vi "Begin.vi"() -> (0 "error out":errorcluster)   [LabVIEW 2013]
doc: "Called before other user functions, this VI is expected to open initial I/O refnums, load in file data, and do all program initialization. Notice that the <B>error out</B> terminal is simply used for data flow. Wiring it to other structures or subVIs ensures that this VI runs first."
uses:
  <vilib>/Rock Robotics/WPI/DriverStation/WPI_DriverStationRobotMode2.ctl
  <vilib>/Rock Robotics/WPI/Joystick/WPI_JoystickDeviceEnum.ctl
  <vilib>/Rock Robotics/SystemInterfaces/DIO/FPGA_DIOPWMChannel.ctl
  <vilib>/Rock Robotics/SystemInterfaces/DIO/FPGA_DIOChannel.ctl
  <vilib>/Rock Robotics/SystemInterfaces/Typedef/FPGA_TypedefDigitalModule.ctl
  Robot Global Data.vi
  <vilib>/Rock Robotics/WPI/RobotDrive/WPI_RobotDriveOpen4MotorWithVictor.vi
  <vilib>/Rock Robotics/WPI/Counter/WPI_CounterDigitalInputToDigitalSource.vi
  <vilib>/Rock Robotics/WPI/Counter/WPI_CounterOpen UpDown Mode.vi
  <vilib>/Rock Robotics/WPI/MotorControl/WPI_MotorControlOpen Victor.vi
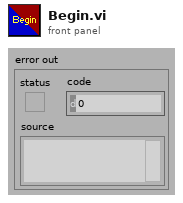
[diagram p1: front panel]
types:
  T1 = typedef "FPGA_DIOPWMChannel.ctl" = enum8{"PWM 1", "PWM 2", "PWM 3", "PWM 4", "PWM 5", "PWM 6", "PWM 7", "PWM 8", "PWM 9", "PWM 10", "Invalid"}
  T2 = typedef "FPGA_TypedefDigitalModule.ctl" = enum16{"Digital Module 1", "Digital Module 2"}
  T3 = typedef "FPGA_DIOChannel.ctl" = enum8{"DIO 1", "DIO 2", "DIO 3", "DIO 4", "DIO 5", "DIO 6", "DIO 7", "DIO 8", "DIO 9", "DIO 10", "DIO 11", "DIO 12", "DIO 13", "DIO 14", "Invalid"}
  T4 = typedef "WPI_JoystickDeviceEnum.ctl" = enum16{"USB 1", "USB 2", "USB 3", "USB 4", "Kinect 1", "Kinect 2"}
  T5 = typedef "WPI_DriverStationRobotMode2.ctl" = enum16{"Autonomous Disabled", "Autonomous Enabled", "Teleop Disabled", "Teleop Enabled", "Timeout", "Finish", "Test Disabled", "Test Enabled"}
  T6 = typedef "WPI_JoystickDevRef.ctl" = cluster{"Device":T4}
  T7 = typedef "WPI_DigitalInputDevRef.ctl" = cluster{"DevStatus":errorcluster, "DIO Channel":T3, "Digital Module":T2}
  T8 = typedef "WPI_MotorControlDeviceRef.ctl" = cluster{"DeviceStatus":errorcluster, "Type":enum16{"PWM", "CAN"}, "PWM":cluster{"Digital Module":T2, "PWM Channel":T1, "DeadBand":T9}, "CAN":cluster{"Device Number":u8, "Control Mode":T10, "Semaphore":T11, "Max Vout":dbl}, "Invert":bool, "TransformRef":T12, "InvTransformRef":T12}
  T9 = typedef "WPI_PWMDeadband.ctl" = cluster{"Name":string, "maxPositivePwm":i32, "minPositivePwm":i32, "centerPwm":i32, "maxNegativePwm":i32, "minNegativePwm":i32, "angularRange":u16}
  T10 = typedef "WPI_CANJaguar_ControlMode.ctl" = enum8{"Percent VBus", "Current", "Speed", "Position", "Voltage"}
  T11 = typedef "Semaphore RefNum" = refnum<k1>
  T12 = typedef "WPI_PWMTransform_ConPane.ctl" = refnum<vi>
  T13 = typedef "WPI_RobotDriveDevRef.ctl" = cluster{"DevStatus":errorcluster, "Motors[]":T8[], "Square Inputs":bool, "Max Output":dbl, "Isochronous":bool}
  T14 = typedef "FPGA_CounterEncoderSourceConvertionLVSourceType.ctl" = cluster{"DevStatus":errorcluster, "AnalogTriggerMode?":bool, "DigitalMode":cluster{"Digital Module":T2, "DIO Channel":T15}, "AnalogTriggerMode":cluster{"AnalogTriggerIndex":T16, "OutputType":T17}}
  T15 = typedef "FPGA_DIODigitalSourceChannel.ctl" = enum8{"DIO 1", "DIO 2", "DIO 3", "DIO 4", "DIO 5", "DIO 6", "DIO 7", "DIO 8", "DIO 9", "DIO 10", "DIO 11", "DIO 12", "DIO 13", "DIO 14", "Disabled"}
  T16 = typedef "FPGA_AnalogTriggerIndex.ctl" = enum8{"Trig 0", "Trig 1", "Trig 2", "Trig 3", "Trig 4", "Trig 5", "Trig 6", "Trig 7", "Invalid"}
  T17 = typedef "FPGA_AnalogTriggerOutType.ctl" = enum16{"InWindow", "TriggerState", "Rising", "Falling"}
  T18 = typedef "WPI_CounterDevRef.ctl" = cluster{"DevStatus":errorcluster, "CntIndex":T19}
  T19 = typedef "FPGA_CounterCtrSystemIndex.ctl" = enum8{"Ctr 0", "Ctr 1", "Ctr 2", "Ctr 3", "Ctr 4", "Ctr 5", "Ctr 6", "Ctr 7", "Invalid"}
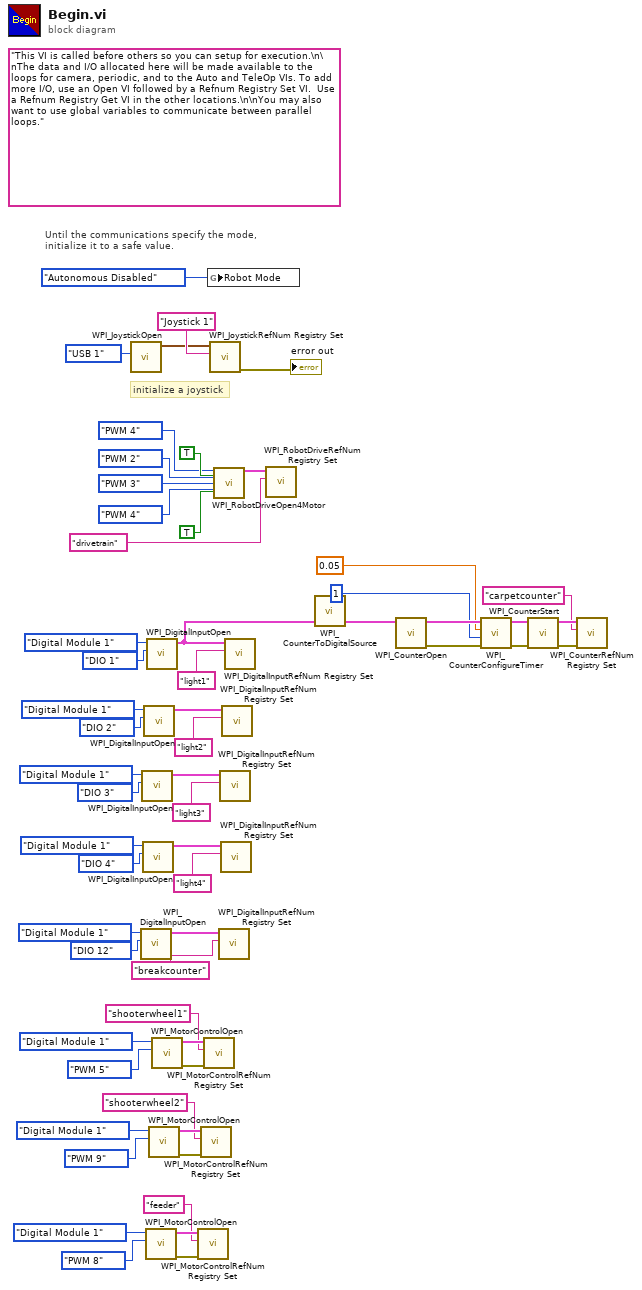
[diagram p0: block diagram]
diagram:
  (unwired) "This VI is called before others so you can setup for execution.\n\nThe data and I/O allocated here will be made available to the loops for camera, periodic, and to the Auto and TeleOp VIs. To add more I/O, use an Open VI followed by a Refnum Registry Set VI.  Use a Refnum Registry Get VI in the other locations.\n\nYou may also want to use global variables to communicate between parallel loops."
  # "initialize a joystick"
  # "Until the communications specify the mode,\ninitialize it to a safe value."
  n1 = call <vilib>:"WPI_JoystickOpen.vi"("JoystickDevice"=WPI_JoystickDeviceEnum."USB 1") -> ("JoystickDevRef"=w56:T6)  [unwired: 10 in]
  n2 = call <vilib>:"WPI_DigitalInputOpen.vi"("DIO Channel"=FPGA_DIOChannel."DIO 12", "Digital Module (Module 1)"=FPGA_TypedefDigitalModule."Digital Module 1") -> ("DigitalInputDevRef"=w30:T7)  [unwired: 8 in, 1 out]
  n3 = call <vilib>:"WPI_DigitalInputOpen.vi"("DIO Channel"=FPGA_DIOChannel."DIO 3", "Digital Module (Module 1)"=FPGA_TypedefDigitalModule."Digital Module 1") -> ("DigitalInputDevRef"=w38:T7)  [unwired: 8 in, 1 out]
  n4 = call <vilib>:"WPI_DigitalInputOpen.vi"("DIO Channel"=FPGA_DIOChannel."DIO 4", "Digital Module (Module 1)"=FPGA_TypedefDigitalModule."Digital Module 1") -> ("DigitalInputDevRef"=w34:T7)  [unwired: 8 in, 1 out]
  n5 = call <vilib>:"WPI_DigitalInputOpen.vi"("DIO Channel"=FPGA_DIOChannel."DIO 2", "Digital Module (Module 1)"=FPGA_TypedefDigitalModule."Digital Module 1") -> ("DigitalInputDevRef"=w42:T7)  [unwired: 8 in, 1 out]
  n6 = call-poly <vilib>:"WPI_MotorControlOpen.vi"("PWM Channel"=FPGA_DIOPWMChannel."PWM 8", "Digital Module (Module 1)"=FPGA_TypedefDigitalModule."Digital Module 1") -> ("error out"=w4:errorcluster, "MotorControlDeviceRef"=w5:T8)  [unwired: 8 in]
  n7 = call <vilib>:"WPI_DigitalInputOpen.vi"("DIO Channel"=FPGA_DIOChannel."DIO 1", "Digital Module (Module 1)"=FPGA_TypedefDigitalModule."Digital Module 1") -> ("DigitalInputDevRef"=w17:T7)  [unwired: 8 in, 1 out]
  n8 = call-poly <vilib>:"WPI_MotorControlOpen.vi"("PWM Channel"=FPGA_DIOPWMChannel."PWM 9", "Digital Module (Module 1)"=FPGA_TypedefDigitalModule."Digital Module 1") -> ("error out"=w10:errorcluster, "MotorControlDeviceRef"=w11:T8)  [unwired: 8 in]
  n9 = call-poly <vilib>:"WPI_MotorControlOpen.vi"("PWM Channel"=FPGA_DIOPWMChannel."PWM 5", "Digital Module (Module 1)"=FPGA_TypedefDigitalModule."Digital Module 1") -> ("error out"=w14:errorcluster, "MotorControlDeviceRef"=w15:T8)  [unwired: 8 in]
  n10 = call <vilib>:"WPI_MotorControlRefNum Registry Set.vi"("error in (no error)"=w4, "refnum name"="feeder", "MotorControlDevRef"=w5) -> ()  [unwired: 7 in, 2 out]
  n11 = call <vilib>:"WPI_MotorControlRefNum Registry Set.vi"("error in (no error)"=w10, "refnum name"="shooterwheel2", "MotorControlDevRef"=w11) -> ()  [unwired: 7 in, 2 out]
  n12 = call <vilib>:"WPI_MotorControlRefNum Registry Set.vi"("error in (no error)"=w14, "refnum name"="shooterwheel1", "MotorControlDevRef"=w15) -> ()  [unwired: 7 in, 2 out]
  n13 = global write "Robot Global Data.vi" "Robot Mode"(WPI_DriverStationRobotMode2."Autonomous Disabled" ("Robot Mode")) -> ()
  n14 = call <vilib>:"WPI_JoystickRefNum Registry Set.vi"("refnum name"="Joystick 1", "JoystickDevRef"=w56) -> ("error out"=→"error out":errorcluster)  [unwired: 8 in, 1 out]
  n15 = call-poly <vilib>:"WPI_RobotDriveOpen4Motor.vi"("Rear Left Motor"=FPGA_DIOPWMChannel."PWM 4", "Rear Right Motor Inverted"=TRUE, "Rear Right Motor"=FPGA_DIOPWMChannel."PWM 2", "Front Left Motor"=FPGA_DIOPWMChannel."PWM 3", "Front Right Motor"=FPGA_DIOPWMChannel."PWM 4", "Front Right Motor Inverted"=TRUE) -> ("RobotDriveDevRef"=w47:T13)  [unwired: 8 in, 1 out]
  n16 = call <vilib>:"WPI_DigitalInputRefNum Registry Set.vi"("refnum name"="breakcounter", "DigitalInputDevRef"=w30) -> ()  [unwired: 8 in, 2 out]
  n17 = call <vilib>:"WPI_DigitalInputRefNum Registry Set.vi"("refnum name"="light3", "DigitalInputDevRef"=w38) -> ()  [unwired: 8 in, 2 out]
  n18 = call <vilib>:"WPI_DigitalInputRefNum Registry Set.vi"("refnum name"="light4", "DigitalInputDevRef"=w34) -> ()  [unwired: 8 in, 2 out]
  n19 = call <vilib>:"WPI_DigitalInputRefNum Registry Set.vi"("refnum name"="light2", "DigitalInputDevRef"=w42) -> ()  [unwired: 8 in, 2 out]
  n20 = call <vilib>:"WPI_DigitalInputRefNum Registry Set.vi"("refnum name"="light1", "DigitalInputDevRef"=w17) -> ()  [unwired: 8 in, 2 out]
  n21 = call <vilib>:"WPI_RobotDriveRefNum Registry Set.vi"("refnum name"="drivetrain", "RobotDriveDevRef"=w47) -> ()  [unwired: 8 in, 2 out]
  n22 = call-poly <vilib>:"WPI_CounterToDigitalSource.vi"("DigitalInputDevRef"=w17) -> ("Digital Source"=w18:T14)  [unwired: 6 in]
  n23 = call-poly <vilib>:"WPI_CounterOpen.vi"("Up Source"=w18) -> ("error out"=w21:errorcluster, "CounterDevRef"=w22:T18)  [unwired: 9 in]
  n24 = call <vilib>:"WPI_CounterConfigureTimer.vi"("error in (no error)"=w21, "Number Samples to Average"=u8 1, "MaxPeriod (sec)"=0.05, "CounterDevRef in"=w22) -> ("error out"=w26:errorcluster, "CounterDevRef out"=w25:T18)  [unwired: 6 in]
  n25 = call <vilib>:"WPI_CounterStart.vi"("error in (no error)"=w26, "CounterDevRef in"=w25) -> ("error out"=w24:errorcluster, "CounterDevRef out"=w23:T18)  [unwired: 8 in]
  n26 = call <vilib>:"WPI_CounterRefNum Registry Set.vi"("error in (no error)"=w24, "refnum name"="carpetcounter", "CounterDevRef"=w23) -> ()  [unwired: 7 in, 2 out]
